vi "Close Pages.vi"(8 "error in (no error)":errorcluster, 11 "Calling VI in":refnum<vi>) -> (0 "error out":errorcluster, 3 "Calling VI out":refnum<vi>)   [LabVIEW 2020, in "Performance Monitor UI.lvlib" / "Configuration.lvlib"]
doc: "Removes the page (and all its different views) from the DCFG Framework.\n_____\nBased on DCFG Project Template 1.0.0.21.\n____\nPeloton Config 1.0.0.2\nCopyright (c) 2022, Peloton"
uses:
  Configuration.lvlib
  Configuration DVR Global.vi
  <vilib>/Peloton/Peloton Config/Libraries/DCFG Framework/Peloton_DCFG Framework.lvlib
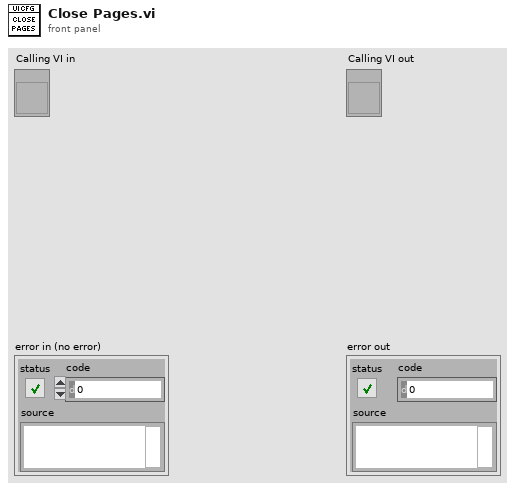
[diagram p1: front panel]
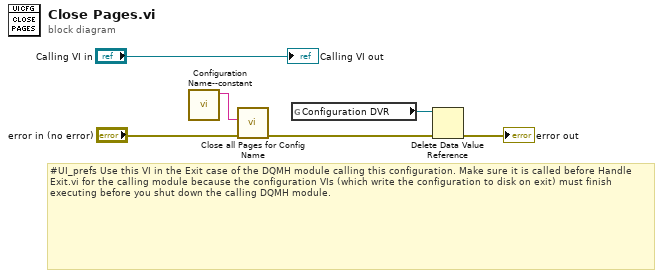
[diagram p0: block diagram]
diagram:
  # "#UI_prefs Use this VI in the Exit case of the DQMH module calling this configuration. Make sure it is called before Handle Exit.vi for the calling module because the configuration VIs (which write the configuration to disk on exit) must finish executing before you shut down the calling DQMH module."
  n1 = call "Configuration Name--constant.vi"() -> ("Configuration Name"=w6:string)  [unwired: 11 in]
  n2 = call <vilib>:"Close all Pages for Config Name.vi"("error in"="error in (no error)", "Configuration Name"=w6) -> ("error out"=w5:errorcluster)  [unwired: 9 in]
  n3 = global read "Configuration DVR Global.vi" "Configuration DVR"() -> (w1:refnum<data-value>)
  n4 = Delete Data Value Reference(data value reference=w1, error in=w5) -> (error out=→"error out":errorcluster)  [unwired: 1 out]
  "Calling VI out" <- "Calling VI in"
